vi "sig.disallow_pause_lua.vi"(5 "LuaVIEW reference":T1) -> (15 "error out":errorcluster)   [LabVIEW 2012]
doc: "Disallow the pause signal. If the pause signal was set prior to calling this function, it will be cleared. This function is required when a task overrides the default handling of pausing using \"handle_pausing\". Alternatively, it can be used to specifically disallow the pause signal but not any of the other signals, e.g. when your task manages some process that can be stopped but must otherwise run continuously. To disable the handling of all signals, use \"begin_protected\" instead. To disallow all manual signals as sent via the Task Manager user interface window but allow programmatic signals, use the \"--#disallow_manual\" preprocessor keyword in the main task script.\nErrors:\nFunction must be called from a task context but was not."
uses:
  typedefs/t_LuaVIEW Reference.ctl
  typedefs/t_LuaVIEW Task Signals.ctl
  typedefs/t_LuaVIEW Task State Methods.ctl
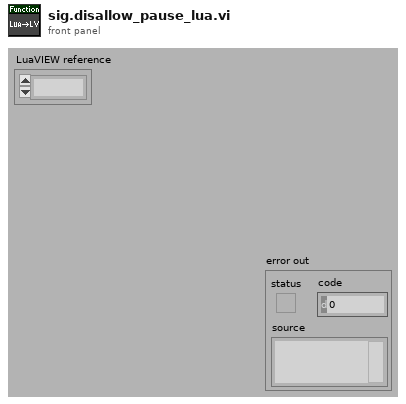
[diagram p1: front panel]
types:
  T1 = typedef "t_LuaVIEW Reference.ctl" = refnum<k1>
  T2 = typedef "t_LuaVIEW Task State Methods.ctl" = enum16{"cleanup", "set initial", "set mode", "set active mode", "set error", "get task info", "get script info", "set signal", "clear signal", "test handled", "test delegated", "test signal", "handle signal", "delegate signal", "allow signal", "disallow signal", "disallow all", "signals?", "delegated signals?", "protection++", "protection--", "protection=0", "message", "next message", "pop message", "message available?", "force stop", "set swap preps", "apply swap preps"}
  T3 = typedef "t_LuaVIEW Task Signals.ctl" = enum32{"resume", "pause", "swap", "stop", "confirm"}
  T4 = typedef "t_LuaVIEW Task State Pane.ctl" = refnum<vi>
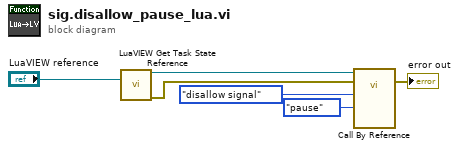
[diagram p0: block diagram]
diagram:
  n1 = call "LuaVIEW Get Task State Reference.vi"("LuaVIEW reference in"="LuaVIEW reference") -> ("task state reference"=w5:T4, "error out"=w1:errorcluster)  [unwired: 12 in, 1 out]
  n2 = call-by-ref "?"(reference=w5, error in=w1, "method"=t_LuaVIEW_Task_State_Methods."disallow signal", "signal"=t_LuaVIEW_Task_Signals."pause") -> (error out=→"error out":errorcluster)  [unwired: 9 in, 6 out]
